vi "GetValueStringFromColor.vi"(10 "Value Width":enum16{"4-bit", "8-bit"}(ring), 11 "Color":u32(colorbox)) -> (3 "Value String":string)   [LabVIEW 2023, in "ArduinoSerialBling.lvlib"]
uses:
  ArduinoSerialBling.lvlib
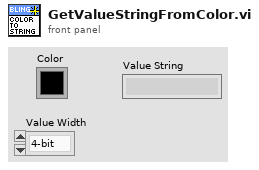
[diagram p1: front panel]
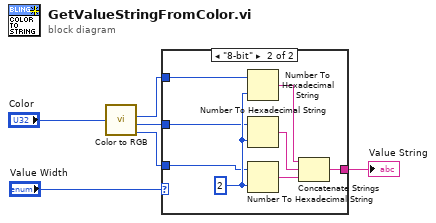
[diagram p0: block diagram]
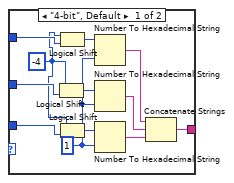
[diagram p2: hidden frame]
diagram:
  n1 = call <vilib>:"Color to RGB.vi"("Color"="Color") -> ("R"=w2:u8, "G"=w3:u8, "B"=w4:u8)  [unwired: 1 out]
  n2 = case shown="\"8-bit\"" "Value Width" {
    tunnel: w2 -> [w13 w25]
    tunnel: w3 -> [w8 w24]
    tunnel: w4 -> [w9 w23]
    tunnel: [w14 w19] -> w6
    frame "4-bit", Default {
      w7 = -4
      w18 = i16 1 ("width (-)")
      n3 = Logical Shift(y=w7, x=w8) -> (x << y=w11:u8)
      n4 = Logical Shift(y=w7, x=w13) -> (x << y=w12:u8)
      n5 = Logical Shift(y=w7, x=w9) -> (x << y=w10:u8)
      n6 = Number To Hexadecimal String(1:w18, 2:w12) -> (0:w17:string)
      n7 = Number To Hexadecimal String(1:w18, 2:w11) -> (0:w16:string)
      n8 = Number To Hexadecimal String(1:w18, 2:w10) -> (0:w15:string)
      n9 = Concatenate Strings(w17, w16, w15) -> (w14:string)
    }
    frame "8-bit" {
      w26 = i16 2 ("width (-)")
      n10 = Number To Hexadecimal String(1:w26, 2:w25) -> (0:w22:string)
      n11 = Number To Hexadecimal String(1:w26, 2:w24) -> (0:w21:string)
      n12 = Number To Hexadecimal String(1:w26, 2:w23) -> (0:w20:string)
      n13 = Concatenate Strings(w22, w21, w20) -> (w19:string)
    }
  }
  "Value String" <- w6
